vi "Compute Friction.vi"(8 "error in (no error)":errorcluster, 9 "gear ratio":dbl=1.0, 10 "qd":dbl, 11 "link in":refnum<class "NI_Robotics_Link.lvclass">) -> (0 "error out":errorcluster, 2 "Friction":dbl, 3 "link out":refnum<class "NI_Robotics_Link.lvclass">)   [LabVIEW 2017, in "NI_Robotics_Link.lvclass"]
uses:
  <vilib>/robotics/Kinematics/Link/NI_Robotics_Link.lvclass
  <vilib>/robotics/Kinematics/Link/NI_Robotics_Link.lvclass/NI_Robotics_Link.ctl
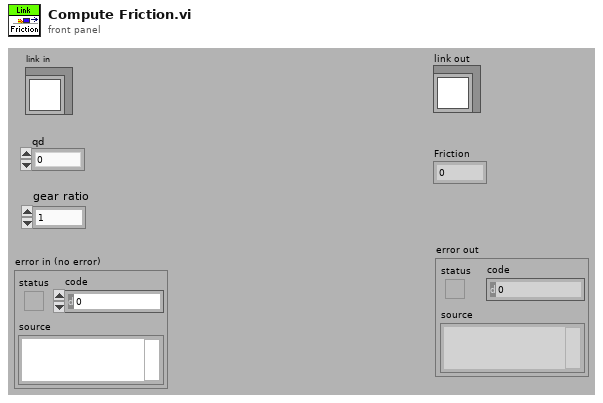
[diagram p1: front panel]
types:
  T1 = cluster{"Positive Movement":dbl, "Negative Movement":dbl}
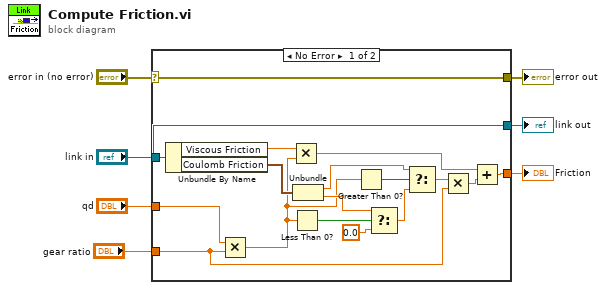
[diagram p0: block diagram]
diagram:
  n1 = case shown="No Error" "error in (no error)" {
    selector: "error in (no error)" -> [w13 w25]
    tunnel: "link in" -> [w14 w26]
    tunnel: "qd" -> [w10 _]
    tunnel: [w16 _] -> w5
    tunnel: [w14 w26] -> w4
    tunnel: [w13 w25] -> w3
    tunnel: "gear ratio" -> [w8 _]
    frame No Error {
      n2 = Unbundle By Name(w14) -> ("Viscous Friction"=w24:dbl, "Coulomb Friction"=w23:T1)
      n3 = Multiply(x=w10, y=w8) -> (x*y=w9:dbl)
      n4 = Multiply(x=w24, y=w9) -> (x*y=w17:dbl)
      n5 = Less Than 0?(x=w9) -> (x < 0?=w21:bool)
      n6 = Unbundle(w23) -> ("Positive Movement"=w20:dbl, "Negative Movement"=w18:dbl)
      n7 = Greater Than 0?(x=w9) -> (x > 0?=w22:bool)
      n8 = Select(t=w18, s=w21, f=0.0) -> (s? t:f=w19:dbl)
      n9 = Select(t=w20, s=w22, f=w19) -> (s? t:f=w12:dbl)
      n10 = Multiply(x=w12, y=w8) -> (x*y=w11:dbl)
      n11 = Add(x=w17, y=w11) -> (x+y=w16:dbl)
    }
    frame Error {
    }
  }
  "link out" <- w4
  "Friction" <- w5
  "error out" <- w3
